vi "UnghiServoGlobal.vi"() -> ()   [LabVIEW 2020]
panel:
  in  "Unghi Servo":dbl(knob) min=0.0 max=165.0 step=5.0 scale=0.0..165.0
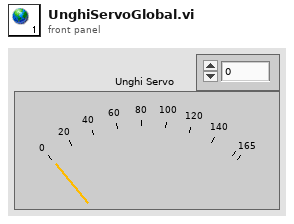
[diagram p1: front panel]
diagram:
